vi "ARC_Queue Flush.vi"(8 "error in (no error)":errorcluster caption="Error In (no error)", 11 "Queue Name(unamed)":string) -> (0 "error out":errorcluster caption="Error Out", 2 "Elements":cluster{"Event":string, "Data":variant}[](array[cluster]))   [LabVIEW 2016]
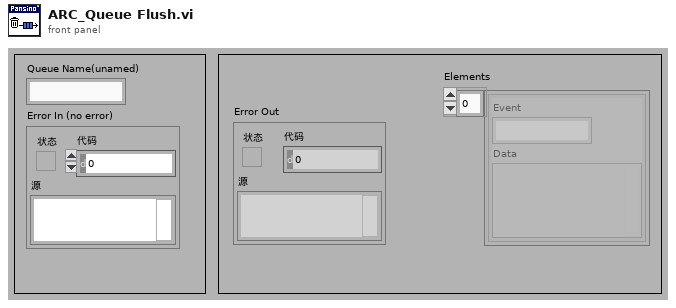
[diagram p1: front panel]
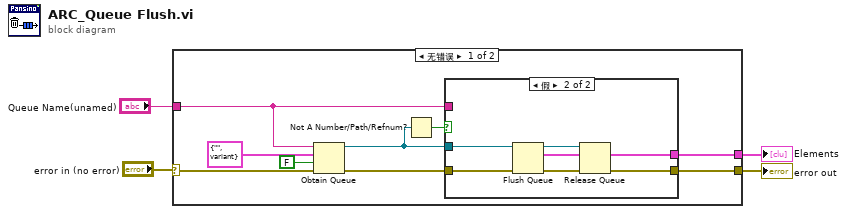
[diagram p0: block diagram]
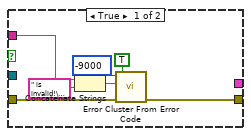
[diagram p2: hidden frame]
diagram:
  n1 = case shown="无错误" "error in (no error)" {
    selector: "error in (no error)" -> [w11 w27]
    tunnel: [w13 w27] -> w3
    tunnel: "Queue Name(unamed)" -> [w7 _]
    tunnel: [w5 _] -> w1
    frame No Error {
      n2 = Obtain Queue(name (unnamed)=w7, element data type=cluster{"Event":string, "Data":variant} {"Event"="", "Data"=variant} ("输出簇"), create if not found? (T)=FALSE ("如未找到是否创建？(T)"), error in (no error)=w11) -> (queue out=w9:refnum<queue>, error out=w12:errorcluster)  [unwired: 1 in, 1 out]
      n3 = Not A Number/Path/Refnum?(number/path/refnum=w9) -> (NaN/Path/Refnum?=w8:bool)
      n4 = case shown="假" w8 {
        tunnel: w12 -> [w17 w25]
        tunnel: [w16 w22] -> w13
        tunnel: [_ w26] -> w5
        tunnel: w9 -> [_ w24]
        tunnel: w7 -> [w14 _]
        frame True {
          n5 = Concatenate Strings(w14, " is invalid!\nEnsure the queue has been created!" ("字符串")) -> (w18:string)
          n6 = call <vilib>:"Error Cluster From Error Code.vi"("show call chain? (False)"=TRUE, "error in (no error)"=w17, "error message (\"\")"=w18, "error code (0)"=-9000) -> ("error out"=w16:errorcluster)  [unwired: 5 in]
        }
        frame False {
          n7 = Flush Queue(queue=w24, error in (no error)=w25) -> (queue out=w21:refnum<queue>, remaining elements=w26:cluster{"Event":string, "Data":variant}[], error out=w23:errorcluster)
          n8 = Release Queue(queue=w21, error in (no error)=w23) -> (error out=w22:errorcluster)  [unwired: 1 in, 2 out]
        }
      }
    }
    frame Error {
    }
  }
  "error out" <- w3
  "Elements" <- w1
